vi "Load Certificates Test.vi"() -> ()   [LabVIEW 2013]
uses:
  SSL_Lib/SSL-Lib/Library Paths.ctl
  SSL_Lib/SSL-Context/SSL Options.ctl
  SSL_Lib/SSL-Lib/SSL-Lib.lvclass
  SSL_Lib/SSL-Context/SSL-Context.lvclass
  SSL_Lib/X509-Cert/X509-Cert.lvclass
panel:
  out "Cert Names":string[](array[string])
  out "Initial Number":i32
  out "Number of Certs":i32
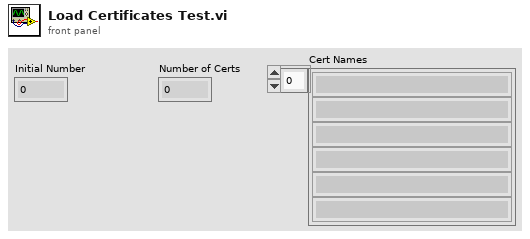
[diagram p1: front panel]
types:
  T1 = typedef "SSL_Lib.lvlib/SSL-Context.lvclass/SSL Options.ctl" = i32
  T2 = typedef "SSL_Lib.lvlib/SSL-Lib.lvclass/Library Paths.ctl" = cluster{"SSL Library Path":path, "Crypto Library Path":path}
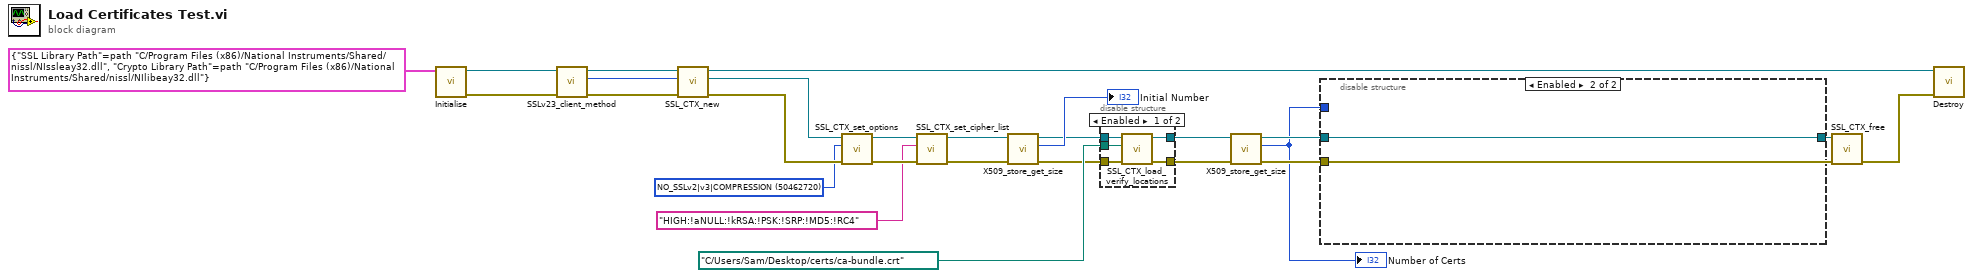
[diagram p0: block diagram]
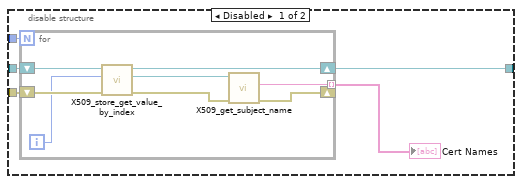
[diagram p2: hidden frame]
diagram:
  w16 = T1 50462720 items=["None"=0, "NO_SSLv2|v3|COMPRESSION"=50462720, "SSL_OP_NO_COMPRESSION"=131072, "SSL_OP_NO_SSLv2"=16777216, "SSL_OP_NO_SSLv3"=33554432, "SSL_OP_NO_TLSv1"=67108864, "SSL_OP_NO_TLSv1_2"=134217728, "SSL_OP_NO_TLSv1_1"=268435456] ("Options")
  n1 = call "Initialise.vi"("Library Paths"=T2 {"SSL Library Path"=path "C:/Program Files (x86)/National Instruments/Shared/nissl/NIssleay32.dll", "Crypto Library Path"=path "C:/Program Files (x86)/National Instruments/Shared/nissl/NIlibeay32.dll"}) -> ("error out"=w22:errorcluster, "SSL-Lib out"=w26:refnum<class "SSL-Lib.lvclass">)  [unwired: 9 in]
  n2 = call "SSLv23_client_method.vi"("error in (no error)"=w22, "SSL-Lib in"=w26) -> ("error out"=w20:errorcluster, "*SSL_Method"=w25:u64, "SSL-Lib out"=w24:refnum<class "SSL-Lib.lvclass">)  [unwired: 7 in]
  n3 = call "SSL_CTX_new.vi"("error in (no error)"=w20, "*SSL_Method"=w25, "SSL-Lib in"=w24) -> ("error out"=w17:errorcluster, "SSL-Context out"=w18:refnum<class "SSL-Context.lvclass">, "SSL-Lib out"=w19:refnum<class "SSL-Lib.lvclass">)  [unwired: 6 in]
  n4 = call "SSL_CTX_set_options.vi"("error in (no error)"=w17, "Options"=w16, "SSL-Context in"=w18) -> ("error out"=w14:errorcluster, "SSL-Context out"=w15:refnum<class "SSL-Context.lvclass">)  [unwired: 7 in]
  n5 = call "SSL_CTX_set_cipher_list.vi"("error in (no error)"=w14, "Cipher List"="HIGH:!aNULL:!kRSA:!PSK:!SRP:!MD5:!RC4", "SSL-Context in"=w15) -> ("error out"=w7:errorcluster, "SSL-Context out"=w8:refnum<class "SSL-Context.lvclass">)  [unwired: 7 in]
  n6 = call "X509_store_get_size.vi"("error in (no error)"=w7, "SSL-Context in"=w8) -> ("error out"=w6:errorcluster, "Size of X509 Store"=→"Initial Number":i32, "SSL-Context out"=w5:refnum<class "SSL-Context.lvclass">)  [unwired: 7 in]
  n7 = disable-structure shown="Enabled" {
    disable-tunnel: [w31 w33] -> w11
    disable-tunnel: [w30 w32] -> w10
    disable-tunnel: w5 -> [w29 w33]
    disable-tunnel: w6 -> [w28 w32]
    disable-tunnel: path "C:/Users/Sam/Desktop/certs/ca-bundle.crt" ("Path to CA bundle") -> [w27 _]
    frame Enabled {
      n8 = call "SSL_CTX_load_verify_locations.vi"("error in (no error)"=w28, "Path to CA bundle"=w27, "SSL-Context in"=w29) -> ("error out"=w30:errorcluster, "SSL-Context out"=w31:refnum<class "SSL-Context.lvclass">)  [unwired: 7 in]
    }
    frame Disabled {
    }
  }
  n9 = call "X509_store_get_size.vi"("error in (no error)"=w10, "SSL-Context in"=w11) -> ("error out"=w4:errorcluster, "Size of X509 Store"=w2:i32, "SSL-Context out"=w3:refnum<class "SSL-Context.lvclass">)  [unwired: 7 in]
  "Number of Certs" <- w2
  n10 = disable-structure shown="Enabled" {
    disable-tunnel: w4 -> [w38 _]
    disable-tunnel: w3 -> [w37 w47]
    disable-tunnel: w2 -> [w36 _]
    disable-tunnel: [w35 w47] -> w1
    frame Disabled {
      n11 = for {
        N: w36 -> [_]
        shift-right: [w41] -> _
        shift-left: w38 -> [w46]
        shift-right: [w40] -> w35
        shift-left: w37 -> [w45]
        tunnel: [w39] -> w34 mode=indexing
        i -> [w42]
        n12 = call "X509_store_get_value_by_index.vi"("error in (no error)"=w46, "Index"=w42, "SSL-Context in"=w45) -> ("error out"=w44:errorcluster, "X509 cert out"=w43:refnum<class "X509-Cert.lvclass">, "SSL-Context out"=w40:refnum<class "SSL-Context.lvclass">)  [unwired: 6 in]
        n13 = call "X509_get_subject_name.vi"("error in (no error)"=w44, "X509-Cert in"=w43) -> ("error out"=w41:errorcluster, "subject name"=w39:string)  [unwired: 7 in, 1 out]
      }
      "Cert Names" <- w34
    }
    frame Enabled {
    }
  }
  n14 = call "SSL_CTX_free.vi"("error in (no error)"=w4, "SSL-Context in"=w1) -> ("error out"=w21:errorcluster)  [unwired: 9 in]
  n15 = call "Destroy.vi"("error in (no error)"=w21, "SSL-Lib in"=w19) -> ()  [unwired: 9 in, 1 out]
